vi "Dipper Fridge Resistance Measurement 1.4.vi"() -> ()   [LabVIEW 2011]
uses:
  <vilib>/express/express arith-compare/Formula/XNode/ExpressFormulaBlockNode.xnode
panel:
  out "XY Graph":cluster{"Y":dbl[], "Y":dbl[]}[](graph)
  out "He Pot Temperature":cluster{dbl[], dbl[]}(graph)
  in  "Sample":bool
  out "Thermometer":bool
  out "Sample":bool
  in  "Timer":bool caption="Reset"
  out "Time Elapsed":string
  out "Output Power":dbl[unit]
  in  "Save":bool
  out "var":i32
  in  "error in (no error) 2":errorcluster
  in  "Output Range":string(combo)
  in  "Heater Power (%)":dbl caption="y"
  out "Heater":bool
  in  "Heater":bool
  out "Boolean":bool
  in  "Power":bool
  in  "Date format (0)":enum16{"short", "long", "abbreviated"}(ring)
  out "Thermometer A":cluster{dbl[], dbl[unit][]}(graph)
  out "size (in bytes)":i64
  out "Thermometer (Ge17035)":cluster{dbl[], dbl[]}(graph)
  in  "File Path":path
  out "current time":timestamp
  out "Number of Data points":i32
  in  "error in (no error)":errorcluster
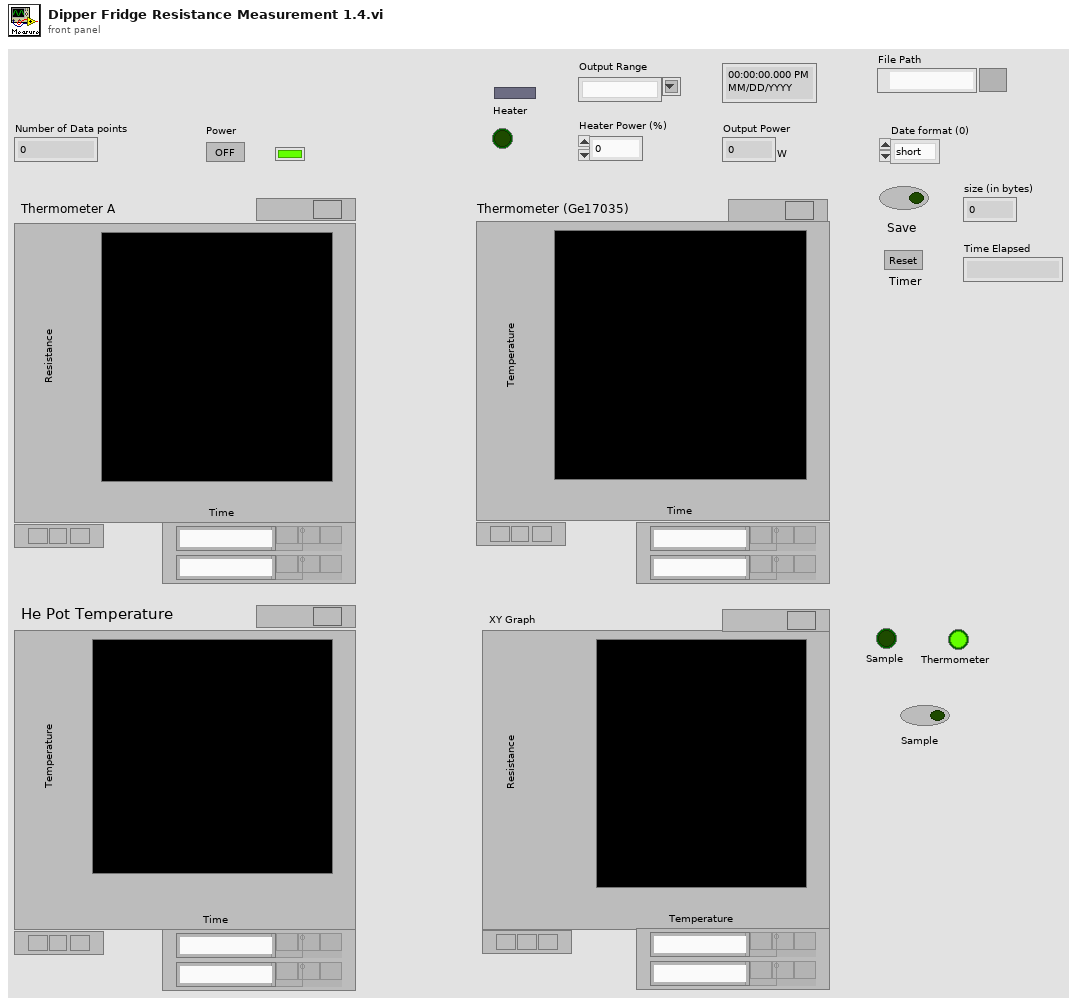
[diagram p1: front panel]
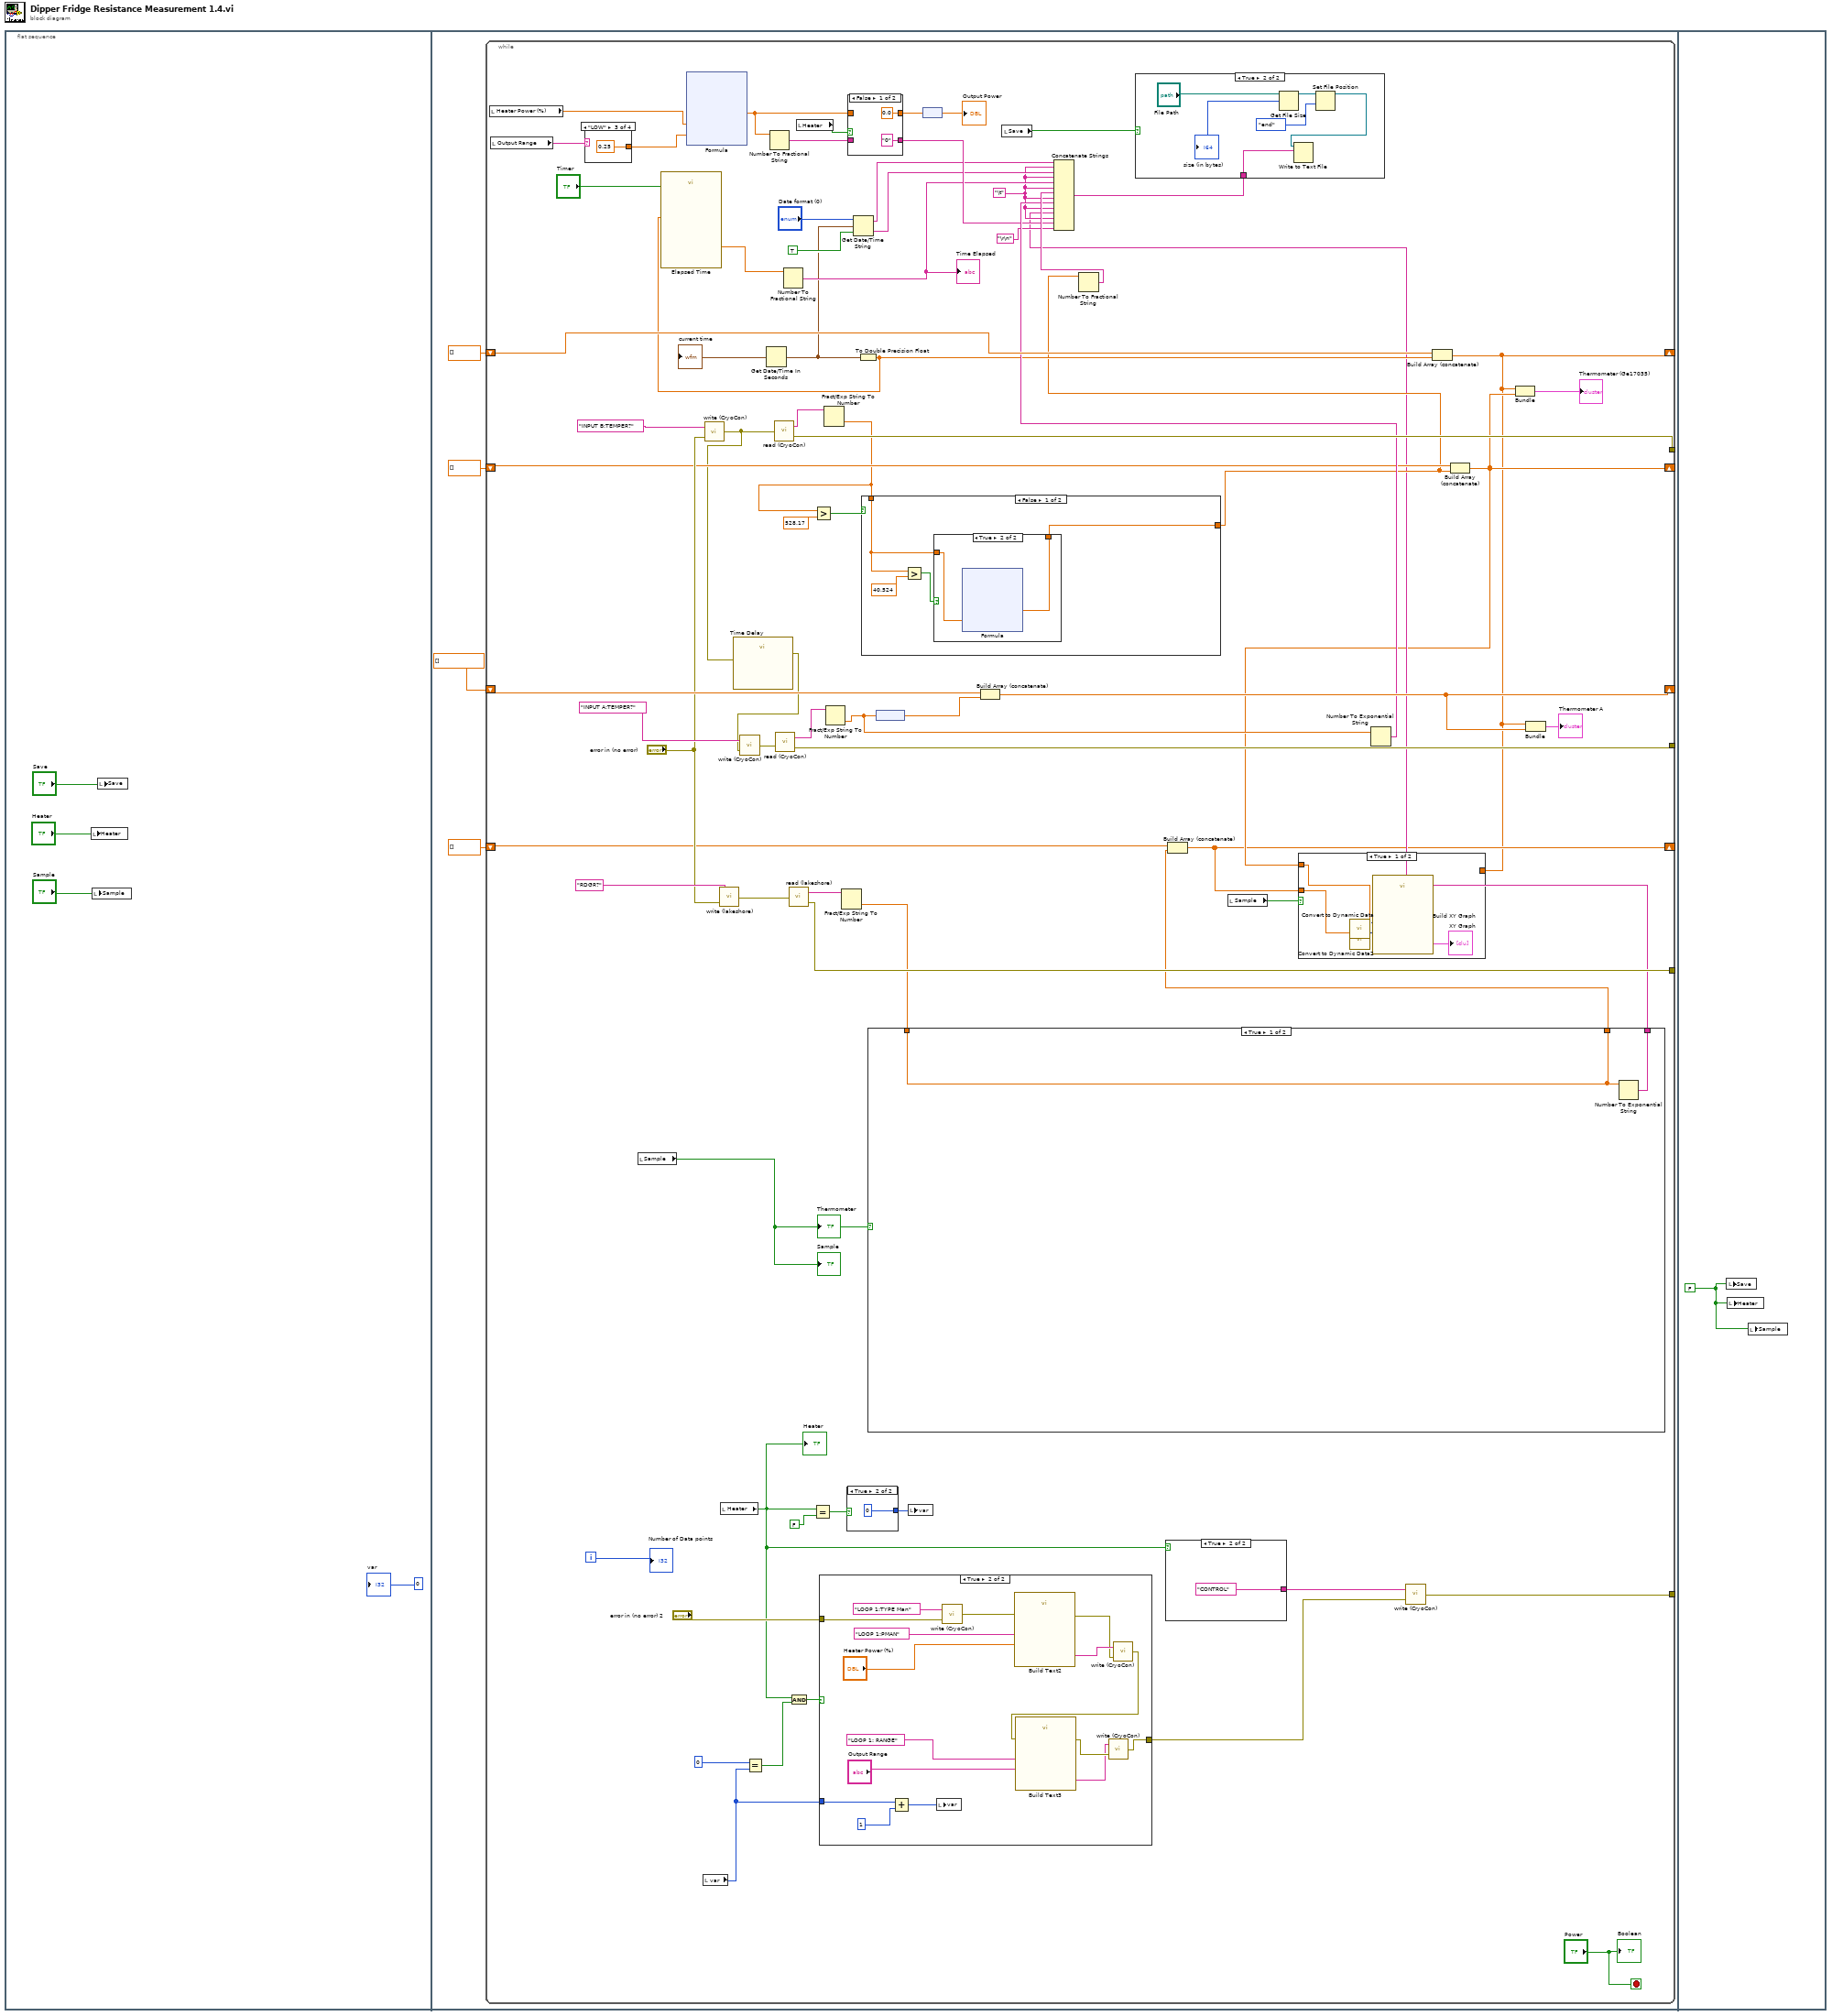
[diagram p0: block diagram]
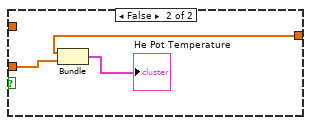
[diagram p2: hidden frame]
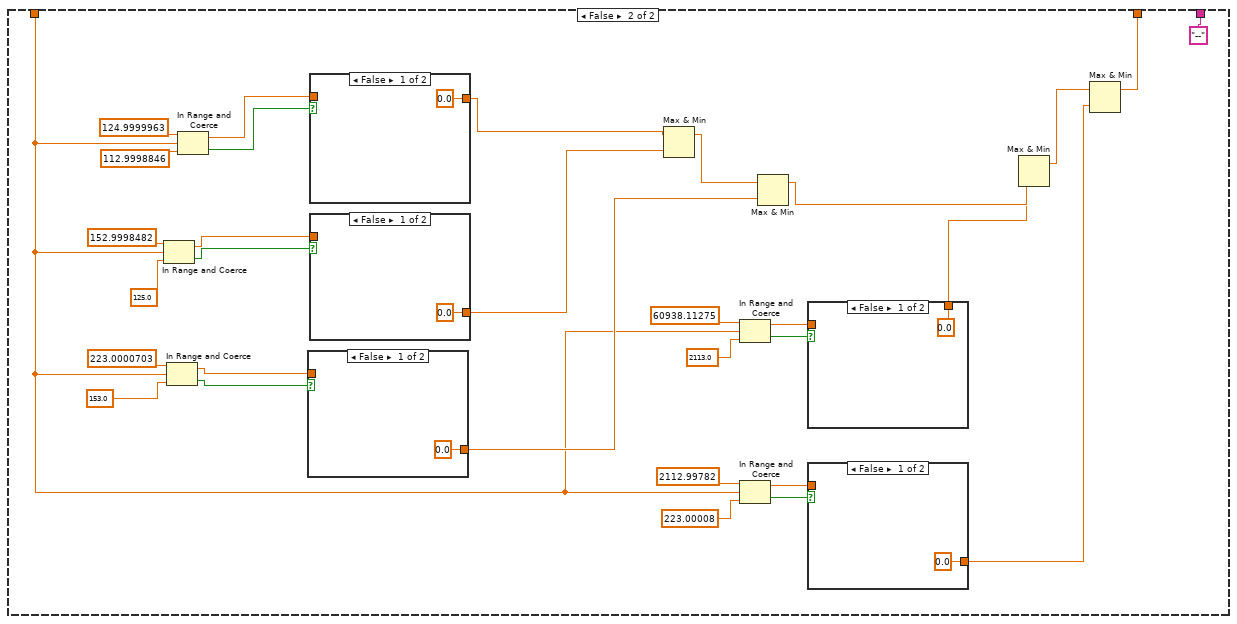
[diagram p3: hidden frame]
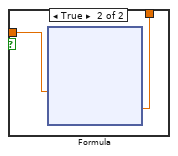
[diagram p4: hidden frame]
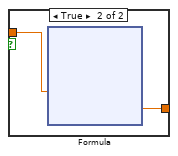
[diagram p5: hidden frame]
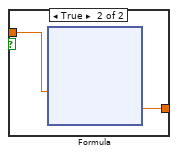
[diagram p6: hidden frame]
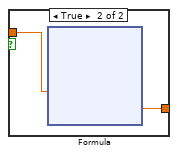
[diagram p7: hidden frame]
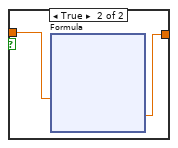
[diagram p8: hidden frame]
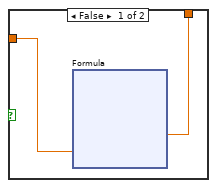
[diagram p9: hidden frame]
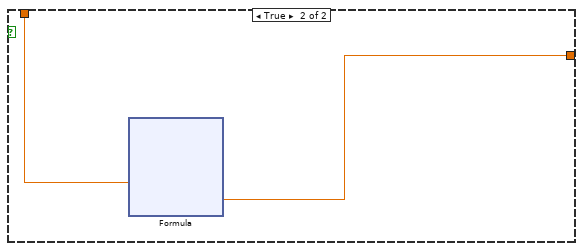
[diagram p10: hidden frame]
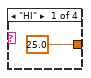
[diagram p12: hidden frame]
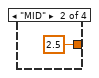
[diagram p13: hidden frame]
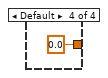
[diagram p14: hidden frame]
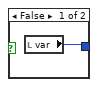
[diagram p15: hidden frame]
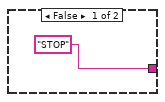
[diagram p17: hidden frame]
diagram:
  n1 = flat-sequence {
    frame #0 {
      n2 = local write "Heater"("Heater") -> ()
      n3 = local write "Sample"("Sample") -> ()
      n4 = local write "Save"("Save") -> ()
      "var" <- 0 ("var")
    }
    frame #1 {
      n5 = while {
        tunnel: [w78] -> _
        tunnel: [w77] -> _
        tunnel: [w73] -> _
        shift-right: [w10] -> _
        shift-left: dbl[] [] -> [w68]
        shift-right: [w64] -> _
        shift-left: dbl[unit][] [] -> [w65]
        shift-right: [w12] -> _
        shift-left: dbl[] [] -> [w57]
        shift-right: [w11] -> _
        shift-left: dbl[] [] -> [w15]
        tunnel: [w9] -> _
        i -> [w70]
        stop <- "Power" stop-if-true
        w23 = "\t"
        n6 = local read "Heater Power (%)"() -> (w42:dbl)
        n7 = local read "Output Range"() -> (w40:string)
        n8 = case shown="\"LOW\"" w40 {
          tunnel: [25.0 ("X2") 2.5 ("X2") 0.25 ("X2") 0.0 ("X2")] -> w41
          frame "HI" {
          }
          frame "MID" {
          }
          frame "LOW" {
          }
          frame Default {
          }
        }
        n9 = local read "Sample"() -> (w14:bool)
        "Sample" <- w14
        "Thermometer" <- w14
        n10 = xnode "Formula"("X1"=w42, "X2"=w41) -> ("Result"=w34:dbl)  [unwired: 1 in, 1 out]
        n11 = local read "var"() -> (w52:i32)
        n12 = call "write (CryoCon).vi"("error in (no error)"="error in (no error)", "write buffer"="INPUT B:TEMPER?") -> ("error out"=w32:errorcluster)
        n13 = call "write (lakeshore).vi"("error in (no error)"="error in (no error)", "write buffer"="RDGR?") -> ("error out"=w72:errorcluster)
        n14 = local read "Heater"() -> (w43:bool)
        "Heater" <- w43
        n15 = call "Time Delay"("error in (no error)"=w32) -> ("error out"=w31:errorcluster)  [unwired: 10 in]
        n16 = call "write (CryoCon).vi"("error in (no error)"=w31, "write buffer"="INPUT A:TEMPER?") -> ("error out"=w79:errorcluster)
        n17 = Equal?(x=0, y=w52) -> (x = y?=w50:bool)
        n18 = Get Date/Time In Seconds() -> (seconds since 1Jan1904=w29:timestamp)
        "current time" <- w29
        n19 = Number To Fractional String(number=w34) -> (F-format string=w38:string)  [unwired: 3 in]
        n20 = call "read (CryoCon).vi"("error in (no error)"=w32) -> ("read buffer"=w75:string, "error out"=w77:errorcluster)
        n21 = call "read (CryoCon).vi"("error in (no error)"=w79) -> ("read buffer"=w76:string, "error out"=w78:errorcluster)
        n22 = call "read (lakeshore).vi"("error in (no error)"=w72) -> ("read buffer"=w74:string, "error out"=w73:errorcluster)
        n23 = And(x=w43, y=w50) -> (x .and. y?=w49:bool)
        n24 = local read "Heater"() -> (w36:bool)
        n25 = Equal?(x=w43, y=FALSE ("Heater")) -> (x = y?=w45:bool)
        n26 = case shown="True" w49 {
          tunnel: [w232 w233] -> w48
          tunnel: "error in (no error) 2" -> [w232 w242]
          tunnel: w52 -> [_ w245]
          frame False {
          }
          frame True {
            n27 = Add(x=w245, y=1) -> (x+y=w243:i32)
            n28 = local write "var"(w243) -> ()
            n29 = call "write (CryoCon).vi"("error in (no error)"=w242, "write buffer"="LOOP 1:TYPE Man") -> ("error out"=w241:errorcluster)
            n30 = call "Build Text2"("x"="LOOP 1:PMAN" ("write buffer"), "y"="Heater Power (%)", "error in (no error)"=w241) -> ("Result"=w238:string, "error out"=w237:errorcluster)  [unwired: 11 in]
            n31 = call "write (CryoCon).vi"("error in (no error)"=w237, "write buffer"=w238) -> ("error out"=w236:errorcluster)
            n32 = call "Build Text3"("x"="LOOP 1: RANGE" ("write buffer"), "y"="Output Range", "error in (no error)"=w236) -> ("Result"=w234:string, "error out"=w235:errorcluster)  [unwired: 11 in]
            n33 = call "write (CryoCon).vi"("error in (no error)"=w235, "write buffer"=w234) -> ("error out"=w233:errorcluster)
          }
        }
        n34 = Fract/Exp String To Number(string=w75) -> (number=w20:dbl)  [unwired: 3 in, 1 out]
        n35 = Greater?(x=w20, y=528.17) -> (0:w21:bool)
        n36 = Fract/Exp String To Number(string=w76) -> (number=w61:dbl)  [unwired: 3 in, 1 out]
        n37 = Fract/Exp String To Number(string=w74) -> (number=w17:dbl)  [unwired: 3 in, 1 out]
        n38 = case shown="True" w45 {
          tunnel: [w220 0] -> w44
          frame False {
            n39 = local read "var"() -> (w220:i32)
          }
          frame True {
          }
        }
        n40 = case shown="False" w36 {
          tunnel: w38 -> [_ w215]
          tunnel: ["0" w215] -> w37
          tunnel: w34 -> [_ w214]
          tunnel: [0.0 ("Result") w214] -> w33
          frame False {
          }
          frame True {
          }
        }
        n41 = Get Date/Time String(date format (0)="Date format (0)", seconds (now)=w29, want seconds? (F)=TRUE) -> (date string=w24:string, time string=w25:string)
        n42 = To Double Precision Float(number=w29) -> (double precision float=w27:dbl)
        n43 = call "Elapsed Time"("Reset"="Timer", "Set Start Time (s)"=w27) -> ("Elapsed Time (s)"=w28:dbl)  [unwired: 10 in, 7 out]
        n44 = Number To Fractional String(number=w28) -> (F-format string=w30:string)  [unwired: 3 in]
        "Time Elapsed" <- w30
        n45 = case shown="False" w21 {
          tunnel: w20 -> [w179 w203]
          tunnel: [w178 w202] -> w19
          frame False {
            n46 = Greater?(x=w179, y=40.524) -> (0:w180:bool)
            n47 = case shown="True" w180 {
              tunnel: [w183 w193] -> w178
              tunnel: w179 -> [w182 w192]
              frame False {
                n48 = xnode "Formula"("X1"=w182) -> ("Result"=w183:dbl)  [unwired: 1 in, 1 out]
              }
              frame True {
                n49 = xnode "Formula"("X1"=w192) -> ("Result"=w193:dbl)  [unwired: 1 in, 1 out]
              }
            }
          }
          frame True {
            n50 = xnode "Formula"("X1"=w203) -> ("Result"=w202:dbl)  [unwired: 1 in, 1 out]
          }
        }
        n51 = case shown="True" w14 {
          tunnel: [w91 "--"] -> w18
          tunnel: w17 -> [w90 w92]
          tunnel: [w90 w94] -> w16
          frame True {
            n52 = Number To Exponential String(number=w90) -> (E-format string=w91:string)  [unwired: 3 in]
          }
          frame False {
            n53 = In Range and Coerce(upper limit=152.9998482, x=w92, lower limit=125.0) -> (coerced(x)=w115:dbl, In Range?=w116:bool)
            n54 = In Range and Coerce(upper limit=223.0000703, x=w92, lower limit=153.0) -> (coerced(x)=w111:dbl, In Range?=w112:bool)
            n55 = In Range and Coerce(upper limit=124.9999963, x=w92, lower limit=112.9998846) -> (coerced(x)=w119:dbl, In Range?=w120:bool)
            n56 = case shown="False" w112 {
              tunnel: w111 -> [_ w147]
              tunnel: [0.0 ("Result") w146] -> w100
              frame False {
              }
              frame True {
                n57 = xnode "Formula"("X1"=w147) -> ("Result"=w146:dbl)  [unwired: 1 in, 1 out]
              }
            }
            n58 = case shown="False" w120 {
              tunnel: w119 -> [_ w169]
              tunnel: [0.0 ("Result") w168] -> w102
              frame False {
              }
              frame True {
                n59 = xnode "Formula"("X1"=w169) -> ("Result"=w168:dbl)  [unwired: 1 in, 1 out]
              }
            }
            n60 = case shown="False" w116 {
              tunnel: w115 -> [_ w158]
              tunnel: [0.0 ("Result") w157] -> w101
              frame False {
              }
              frame True {
                n61 = xnode "Formula"("X1"=w158) -> ("Result"=w157:dbl)  [unwired: 1 in, 1 out]
              }
            }
            n62 = Max & Min(x=w102, y=w101) -> (max(x,y)=w99:dbl)  [unwired: 1 out]
            n63 = In Range and Coerce(upper limit=60938.11275, x=w92, lower limit=2113.0) -> (coerced(x)=w103:dbl, In Range?=w104:bool)
            n64 = In Range and Coerce(upper limit=2112.99782, x=w92, lower limit=223.00008) -> (coerced(x)=w107:dbl, In Range?=w108:bool)
            n65 = Max & Min(x=w99, y=w100) -> (max(x,y)=w98:dbl)  [unwired: 1 out]
            n66 = case shown="False" w104 {
              tunnel: w103 -> [_ w125]
              tunnel: [0.0 ("Result") w124] -> w97
              frame False {
              }
              frame True {
                n67 = xnode "Formula"("X1"=w125) -> ("Result"=w124:dbl)  [unwired: 1 in, 1 out]
              }
            }
            n68 = case shown="False" w108 {
              tunnel: w107 -> [_ w136]
              tunnel: [0.0 ("Result") w135] -> w95
              frame False {
              }
              frame True {
                n69 = xnode "Formula"("X1"=w136) -> ("Result"=w135:dbl)  [unwired: 1 in, 1 out]
              }
            }
            n70 = Max & Min(x=w98, y=w97) -> (max(x,y)=w96:dbl)  [unwired: 1 out]
            n71 = Max & Min(x=w96, y=w95) -> (max(x,y)=w94:dbl)  [unwired: 1 out]
          }
        }
        n72 = node(w61) -> (w66:dbl[unit])
        n73 = local write "var"(w44) -> ()
        n74 = node(w33) -> (→"Output Power":dbl[unit])
        n75 = Build Array (concatenate)(w65, w66) -> (w64:dbl[unit][])
        n76 = local read "Save"() -> (w47:bool)
        n77 = Number To Fractional String(number=w19) -> (F-format string=w60:string)  [unwired: 3 in]
        n78 = case shown="True" w43 {
          tunnel: ["STOP" ("write buffer") "CONTROL" ("write buffer")] -> w54
          frame False {
          }
          frame True {
          }
        }
        n79 = Build Array (concatenate)(w15, w16) -> (w11:dbl[])
        n80 = local read "Sample"() -> (w13:bool)
        n81 = Number To Exponential String(number=w61) -> (E-format string=w59:string)  [unwired: 3 in]
        n82 = Concatenate Strings(w24, w23, w25, w23, w30, w23, w60, w23, w59, w23, w18, w23, w37, "\r\n") -> (w67:string)
        n83 = case shown="True" w47 {
          tunnel: w67 -> [_ w256]
          frame False {
          }
          frame True {
            n84 = Get File Size(file="File Path") -> (refnum out=w254:refnum<file>, size (in bytes)=→"size (in bytes)":i64)  [unwired: 1 in, 1 out]
            n85 = Set File Position(refnum=w254, from (0:start)=enum16{"start", "end", "current"}."end") -> (refnum out=w253:refnum<file>)  [unwired: 2 in, 1 out]
            n86 = Write to Text File(file (use dialog)=w253, text=w256) -> ()  [unwired: 2 in, 3 out]
          }
        }
        n87 = call "write (CryoCon).vi"("error in (no error)"=w48, "write buffer"=w54) -> ("error out"=w9:errorcluster)
        n88 = Build Array (concatenate)(w68, w27) -> (w10:dbl[])
        n89 = Build Array (concatenate)(w57, w19) -> (w12:dbl[])
        n90 = case shown="True" w13 {
          tunnel: w12 -> [w85 _]
          tunnel: w11 -> [w83 w89]
          tunnel: w10 -> [_ w88]
          frame True {
            n91 = call "Convert to Dynamic Data"("Array"=w85) -> ("Dynamic Data Type"=w84:dynamicdata)  [unwired: 3 in]
            n92 = call "Convert to Dynamic Data2"("Array"=w83) -> ("Dynamic Data Type"=w82:dynamicdata)  [unwired: 3 in]
            n93 = call "Build XY Graph"("Y Input"=w82, "X Input"=w84) -> ("XY Graph"=→"XY Graph":cluster{"Y":dbl[], "Y":dbl[]}[])  [unwired: 3 in, 6 out]
          }
          frame False {
            n94 = Bundle(w88, w89) -> (→"He Pot Temperature":cluster{dbl[], dbl[]})  [unwired: 1 in]
          }
        }
        n95 = Bundle(w10, w12) -> (→"Thermometer (Ge17035)":cluster{dbl[], dbl[]})  [unwired: 1 in]
        n96 = Bundle(w10, w64) -> (→"Thermometer A":cluster{dbl[], dbl[unit][]})  [unwired: 1 in]
        "Number of Data points" <- w70
        "Boolean" <- "Power"
      }
    }
    frame #2 {
      w257 = FALSE ("Save")
      n97 = local write "Save"(w257) -> ()
      n98 = local write "Heater"(w257) -> ()
      n99 = local write "Sample"(w257) -> ()
    }
  }
